vi "transmit additional endpoints.vi"(11 "Oauth2.GitHub":refnum<class "Oauth2.GitHub.lvclass">) -> (2 "Additional Endpoints":string[](array[string]))   [LabVIEW 2013, in "Oauth2.GitHub.lvclass"]
uses:
  Oauth2.GitHub.lvclass
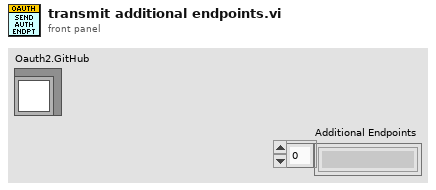
[diagram p1: front panel]
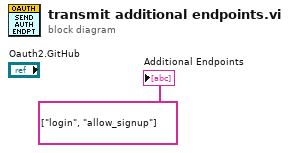
[diagram p0: block diagram]
diagram:
  "Additional Endpoints" <- string[] ["login", "allow_signup"] ("Additional Endpoints")
